vi "Example4-Text.vi"() -> ()   [LabVIEW 2020, in "LcPictureBox.lvclass"]
uses:
  <userlib>/_LabVIEWCommon/LcPictureBox_class/LcPictureBox.lvclass
  System.Windows.Forms
  <userlib>/_LabVIEWCommon/LcPictureBox_class/SmoothingMode.ctl
  System.Drawing
panel:
  in  "PictureBox 1":refnum<k24>(container)
  in  "ZoomFactor":dbl=0.5
  out "error out":errorcluster
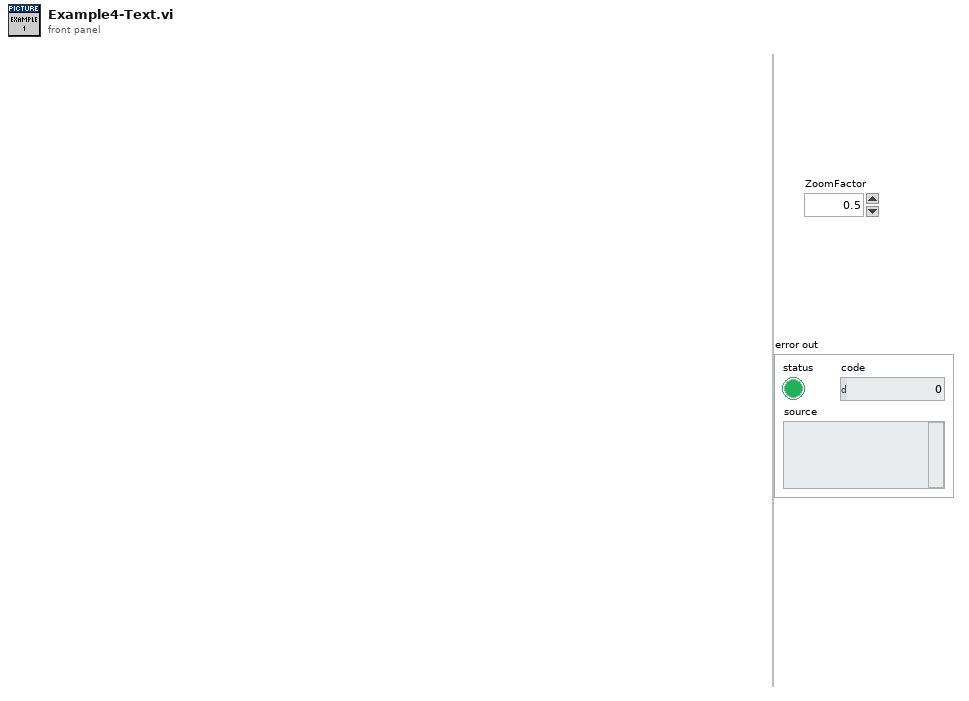
[diagram p1: front panel]
types:
  T1 = cluster{"X":sgl, "Y":sgl, "Width":sgl, "Height":sgl}
  T2 = cluster{"horizontal":enum16{"Left", "Center", "Right"}, "vertical":enum16{"Top", "Center", "Bottom"}}
  T3 = typedef "LcPictureBox.lvclass/SmoothingMode.ctl" = enum16{"None", "HighSpeed", "HighQuality", "AntiAlias"}
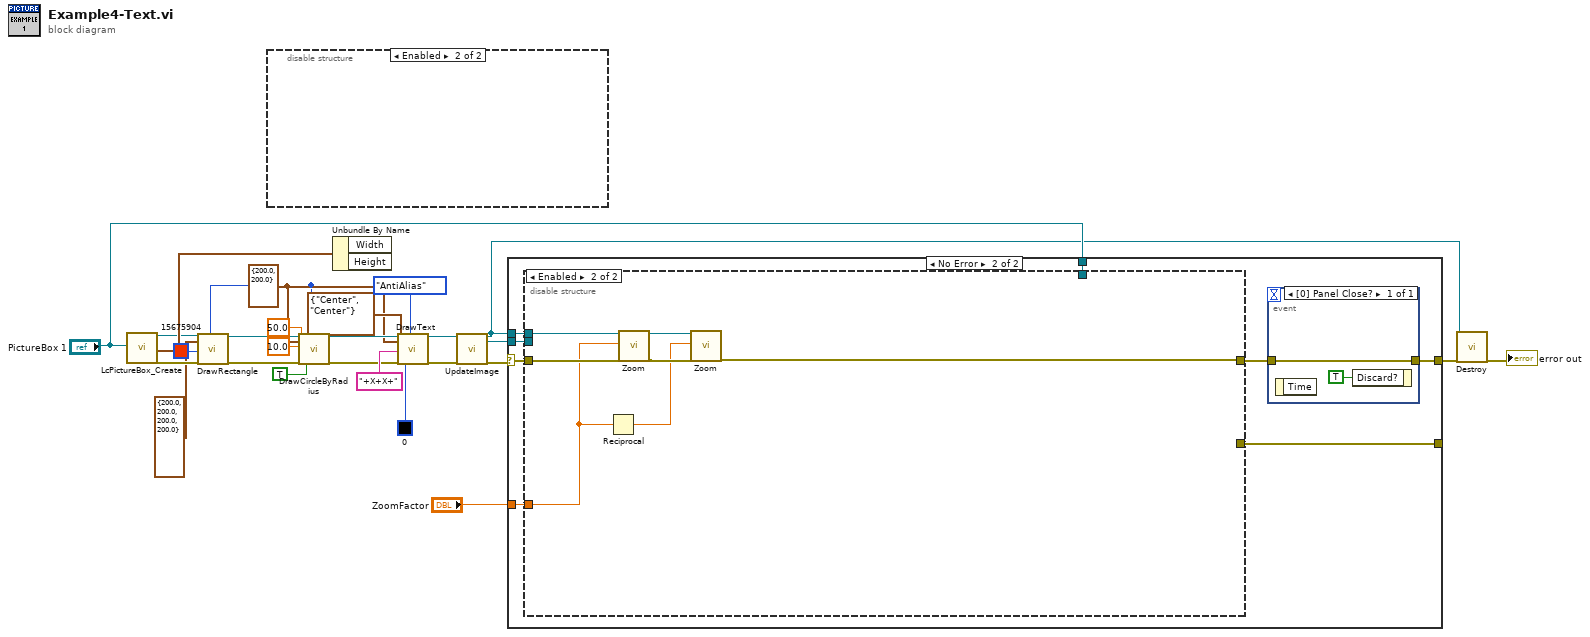
[diagram p0: block diagram]
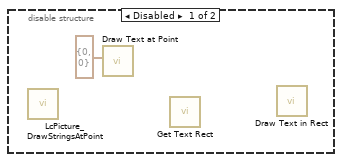
[diagram p2: hidden frame]
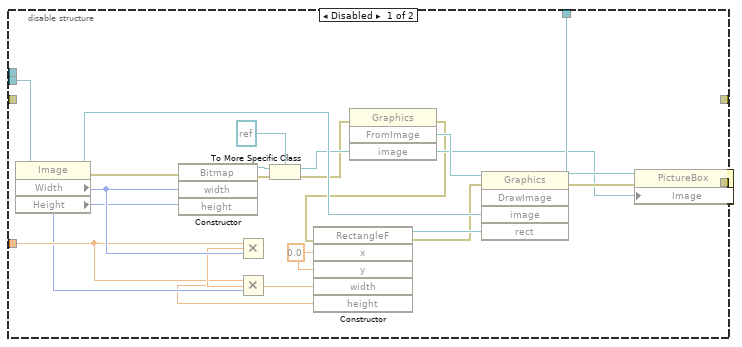
[diagram p4: hidden frame]
diagram:
  w5 = SmoothingMode."AntiAlias" ("SmoothingMode(None)")
  w15 = cluster{"X":sgl, "Y":sgl} {"X"=200.0, "Y"=200.0} ("Origin")
  n1 = call <userlib>:"LcPictureBox_Create.vi"("PictureBox"="PictureBox 1") -> ("reference out"=w10:refnum<class "LcPictureBox.lvclass">, "ImageSizeUsed"=w26:cluster{"Width":i32, "Height":i32}, "Error Out"=w23:errorcluster)  [unwired: 16 in]
  n2 = call-dynamic "DrawRectangle.vi"("reference in"=w10, "Rectangle"=T1 {"X"=200.0, "Y"=200.0, "Width"=200.0, "Height"=200.0}, "Color(Black)"=u32 15675904, "Error In"=w23, "SmoothingMode(None)"=w5) -> ("reference out"=w9:refnum<class "LcPictureBox.lvclass">, "Error Out"=w11:errorcluster)  [unwired: 13 in]
  n3 = disable-structure shown="Enabled" {
    frame Disabled {
      n4 = call <userlib>:"LcPicture_DrawStringsAtPoint.vi"() -> ()  [unwired: 18 in, 2 out]
      n5 = call <vilib>:"Draw Text at Point.vi"("origin"=cluster{"x":i16, "y":i16} {"x"=0, "y"=0}) -> ()  [unwired: 9 in, 2 out]
      n6 = call <vilib>:"Get Text Rect.vi"() -> ()  [unwired: 9 in, 1 out]
      n7 = call <vilib>:"Draw Text in Rect.vi"() -> ()  [unwired: 11 in, 1 out]
    }
    frame Enabled {
    }
  }
  n8 = call-dynamic "DrawCircleByRadius.vi"("reference in"=w9, "Center"=w15, "Radius"=sgl 10.0, "Alpha(100%)"=50.0, "Error In"=w11, "Fill(False)"=TRUE, "SmoothingMode(AntiAlias)"=w5) -> ("reference out"=w16:refnum<class "LcPictureBox.lvclass">, "Error Out"=w17:errorcluster)  [unwired: 11 in]
  n9 = Unbundle By Name(w26) -> ()  [unwired: 2 out]
  n10 = call-dynamic "DrawText.vi"("reference in"=w16, "Origin"=w15, "Alignment(Left,Top)"=T2 {"horizontal"=enum."Center", "vertical"=enum."Center"}, "Text"="+X+X+", "Error In"=w17, "Color(Black)"=u32 0, "SmoothingMode(AntiAlias)"=w5) -> ("reference out"=w21:refnum<class "LcPictureBox.lvclass">, "Error Out"=w20:errorcluster)  [unwired: 11 in]
  n11 = call-dynamic "UpdateImage.vi"("reference in"=w21, "Error In"=w20) -> ("reference out"=w1:refnum<class "LcPictureBox.lvclass">, "ImageUsed"=w4:refnum<k24>, "Error Out"=w19:errorcluster)  [unwired: 14 in, 1 out]
  n12 = case shown="No Error" w19 {
    selector: w19 -> [w28 w31]
    tunnel: [w28 w36] -> w24
    tunnel: w4 -> [_ w35]
    tunnel: "PictureBox 1" -> [_ w34]
    tunnel: "ZoomFactor" -> [_ w33]
    tunnel: [_ w32] -> _
    tunnel: w1 -> [_ w29]
    frame Error {
    }
    frame No Error {
      n13 = disable-structure shown="Enabled" {
        disable-tunnel: w35 -> [w57 _]
        disable-tunnel: w34 -> [w49 _]
        disable-tunnel: w33 -> [w44 w58]
        disable-tunnel: [w37 _] -> w32
        disable-tunnel: w31 -> [_ w64]
        disable-tunnel: [_ w61] -> w30
        disable-tunnel: w29 -> [_ w63]
        frame Disabled {
          w51 = sgl 0.0 ("x")
          n14 = property class="Image"(reference=w57) -> (reference out=w48:refnum<k24>, error out=w41:errorcluster, "Width"=w46:i32, "Height"=w43:i32)  [unwired: 1 in]
          n15 = constructor class="Bitmap"(error in=w41, "width"=w46, "height"=w43) -> (reference out=w55:refnum<k24>, error out=w54:errorcluster)  [unwired: 2 in, 3 out]
          n16 = Multiply(x=w44, y=w46) -> (x*y=w45:dbl)
          n17 = Multiply(x=w44, y=w43) -> (x*y=w42:dbl)
          n18 = To More Specific Class(target class=refnum<k24> refnum, reference=w55, error in=w54) -> (specific class reference=w47:refnum<k24>, error out=w40:errorcluster)
          n19 = invoke class="Graphics" method="FromImage"(error in=w40, "image"=w47) -> (error out=w39:errorcluster, "FromImage"=w53:refnum<k24>)  [unwired: 2 in, 2 out]
          n20 = constructor class="RectangleF"(error in=w39, "x"=w51, "y"=w51, "width"=w45, "height"=w42) -> (reference out=w52:refnum<k24>, error out=w38:errorcluster)  [unwired: 2 in, 5 out]
          n21 = invoke class="Graphics" method="DrawImage"(reference=w53, error in=w38, "image"=w48, "rect"=w52) -> (error out=w50:errorcluster)  [unwired: 1 in, 4 out]
          n22 = property class="PictureBox"(reference=w49, error in=w50, "Image"=w47) -> (error out=w37:errorcluster)  [unwired: 1 out]
        }
        frame Enabled {
          n23 = Reciprocal(x=w58) -> (1/x=w59:dbl)
          n24 = call-dynamic "Zoom.vi"("reference in"=w63, "ZoomFactor"=w58, "Error In"=w64) -> ("reference out"=w60:refnum<class "LcPictureBox.lvclass">, "Error Out"=w62:errorcluster)  [unwired: 13 in, 2 out]
          n25 = call-dynamic "Zoom.vi"("reference in"=w60, "ZoomFactor"=w59, "Error In"=w62) -> ("Error Out"=w61:errorcluster)  [unwired: 13 in, 3 out]
        }
      }
      n26 = event shown="[0] Panel Close?" {
        selector: _ -> [_]
        dyn-events: _ -> [_]
        timeout: _ -> [_]
        tunnel: w30 -> [w65]
        tunnel: [w65] -> w36
        event Panel Close? {
          n27 = event-data() -> ()  [unwired: 1 in, 1 out]
          n28 = event-data("Discard?"=TRUE) -> ()  [unwired: 1 in, 1 out]
        }
      }
    }
  }
  n29 = call-dynamic "Destroy.vi"("reference in"=w1, "Error In"=w24) -> ("Error Out"=→"error out":errorcluster)  [unwired: 16 in, 1 out]
